vi "Create AI Vrms Mode.vi"(7 "mode settings":variant, 8 "error in":errorcluster, 9 "number of channels":i32, 10 "channel settings":T1[](array[typedef]), 11 "ai vrms mode in":refnum<class "Analog Input Vrms Mode.lvclass">) -> (0 "error out":errorcluster, 1 "channels":refnum<class "AI Channel.lvclass">[](array[class]), 3 "ai vrms mode out":refnum<class "Analog Input Vrms Mode.lvclass">)   [LabVIEW 2017, in "Scan Engine Scripting.lvlib" / "Analog Input Vrms Mode.lvclass"]
uses:
  Analog Input Vrms Mode.lvclass
  C:/dev/github.com/debryant/niveristand-scan-engine-ethercat-custom-device/Custom Device Source/Scripting/Modules/Mode Classes/Analog Input Mode/Analog Input Vrms Mode/Analog Input Mode.lvclass
  Channel Classes/AI Channel/AI Channel.lvclass
  Controls/analog channel settings.ctl
  Analog Input Mode/Analog Input Vrms Mode/Analog Input Mode.lvclass
  Scan Engine Scripting.lvlib
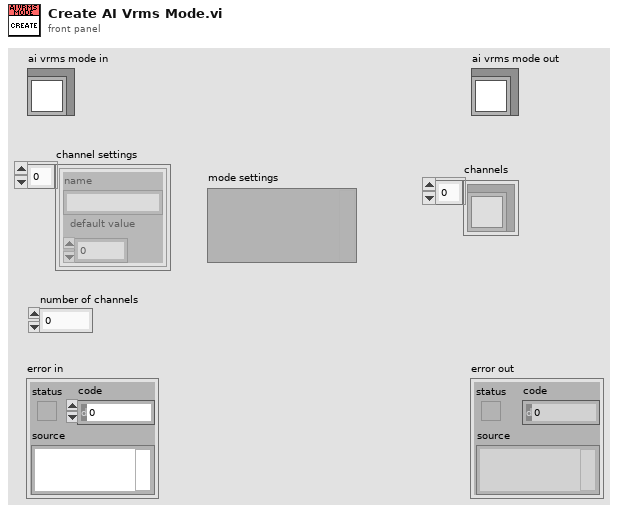
[diagram p1: front panel]
types:
  T1 = typedef "Scan Engine Scripting.lvlib/analog channel settings.ctl" = cluster{"name":string, "default value":dbl}
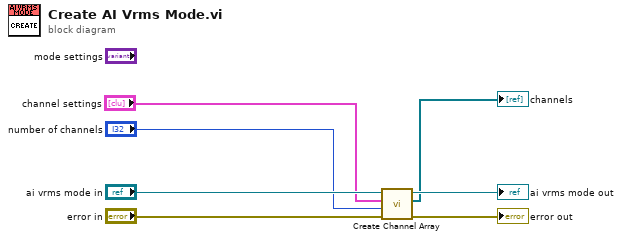
[diagram p0: block diagram]
diagram:
  n1 = call "Create Channel Array.vi"("error in"="error in", "expected channel count"="number of channels", "channel settings"="channel settings", "analog input mode in"="ai vrms mode in") -> ("error out"=→"error out":errorcluster, "channels"=→"channels":refnum<class "AI Channel.lvclass">[], "analog input mode out"=→"ai vrms mode out":refnum<class "Analog Input Vrms Mode.lvclass">)  [unwired: 5 in]
